vi "Corr Get Example Corrections Folder.vi"() -> (1 "corrections path":path, 2 "transducers path":path, 3 "digitizer path":path)   [LabVIEW 2020]
doc: "Returns folder path with example correction datasets."
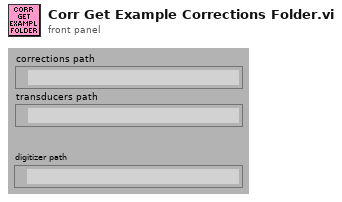
[diagram p1: front panel]
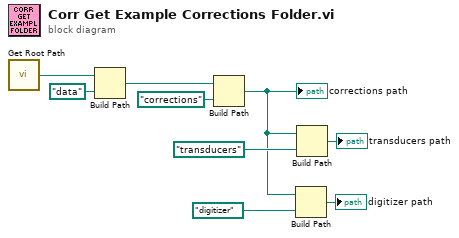
[diagram p0: block diagram]
diagram:
  n1 = call "Get Root Path.vi"() -> ("root path"=w9:path)
  n2 = Build Path(base path=w9, name or relative path=path "data") -> (appended path=w7:path)
  n3 = Build Path(base path=w7, name or relative path=path "corrections") -> (appended path=w1:path)
  "corrections path" <- w1
  n4 = Build Path(base path=w1, name or relative path=path "digitizer") -> (appended path=→"digitizer path":path)
  n5 = Build Path(base path=w1, name or relative path=path "transducers") -> (appended path=→"transducers path":path)
